vi "Reset Analysis ROI.vi"(11 "Analysis Graph in":refnum<class "Graph with Analysis Controls.lvclass">) -> (3 "Analysis Graph out":refnum<class "Graph with Analysis Controls.lvclass">)   [LabVIEW 2023, in "Graph with Analysis Controls.lvclass"]
uses:
  Graph with Analysis Controls.lvclass
  Series Graph/Graph with Series View.lvclass/Graph with Series View.ctl
  Graph with Analysis Controls.lvclass/Graph with Analysis Controls.ctl
  Base Graph/Base Graph.lvclass/Base Graph.ctl
  Get Analysis ROI.vi
  Series Graph/Get Series Graph.vi
  Base Graph/Get ROI X-Y.vi
  Series Graph/Graph with Series View.lvclass
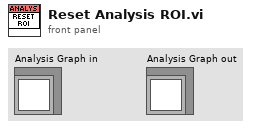
[diagram p1: front panel]
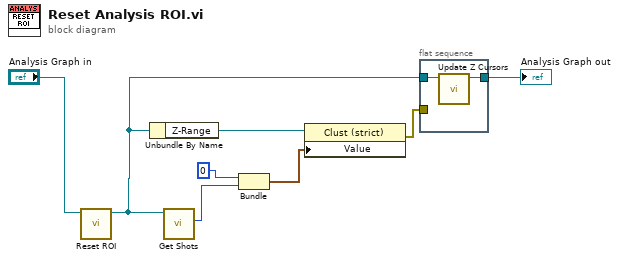
[diagram p0: block diagram]
diagram:
  n1 = call-dynamic "Reset ROI.vi"("Section Graph. in"="Analysis Graph in") -> ("Section Graph. out"=w2:refnum<class "Graph with Analysis Controls.lvclass">)  [unwired: 10 in]
  n2 = Unbundle By Name(w2) -> ("Z-Range"=w6:refnum<vi>)
  n3 = call "Get Shots.vi"("Series Graph in"=w2) -> ("Shots"=w5:u32)  [unwired: 9 in, 1 out]
  n4 = Bundle(0, "Shots"=w5) -> (w3:cluster{i32, "Shots":u32})  [unwired: 1 in]
  n5 = property class="Clust (strict)"(reference=w6, "Value"=w3) -> (error out=w1:errorcluster)  [unwired: 1 in, 1 out]
  n6 = flat-sequence {
    tunnel: [w10] -> w7
    tunnel: w2 -> [w9]
    tunnel: w1 -> [_]
    frame #0 {
      n7 = call "Update Z Cursors.vi"("Analysis Graph in"=w9) -> ("Analysis Graph out"=w10:refnum<class "Graph with Analysis Controls.lvclass">)  [unwired: 10 in]
    }
  }
  "Analysis Graph out" <- w7
